vi "Obtain Message Queue.vi"(8 "error in (no error)":errorcluster, 11 "name (unnamed)":string) -> (0 "error out":errorcluster, 3 "Message Queue":refnum<queue>)   [LabVIEW 2014, in "UI_ProgressDlg.lvlib" / "UI_ProgressDlg.lvclass"]
doc: "Create a queue with the Message Cluster data type."
uses:
  UI_ProgressDlg.lvclass
  Message Cluster.ctl
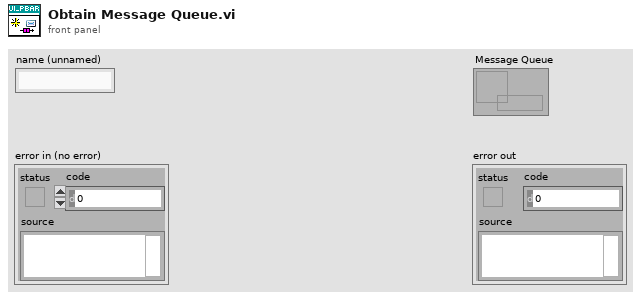
[diagram p1: front panel]
types:
  T1 = typedef "UI_ProgressDlg.lvlib/UI_ProgressDlg.lvclass/Message Cluster.ctl" = cluster{"Message":string, "Message Data":variant}
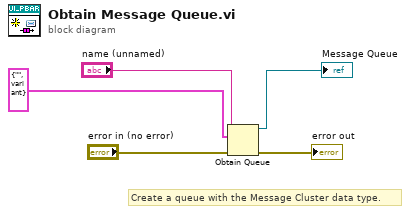
[diagram p0: block diagram]
diagram:
  # "Create a queue with the Message Cluster data type."
  n1 = Obtain Queue(name (unnamed)="name (unnamed)", element data type=T1 {"Message"="", "Message Data"=variant} ("Message Cluster"), error in (no error)="error in (no error)") -> (queue out=→"Message Queue":refnum<queue>, error out=→"error out":errorcluster)  [unwired: 2 in, 1 out]
